vi "Database.Main-CheckStatus.vi"(8 "error in":errorcluster) -> (0 "error out":errorcluster)   [LabVIEW 2016]
uses:
  CheckStatusData.ctl
  Database.Main.Action.ctl
panel:
  in  "CheckStatusData":T1
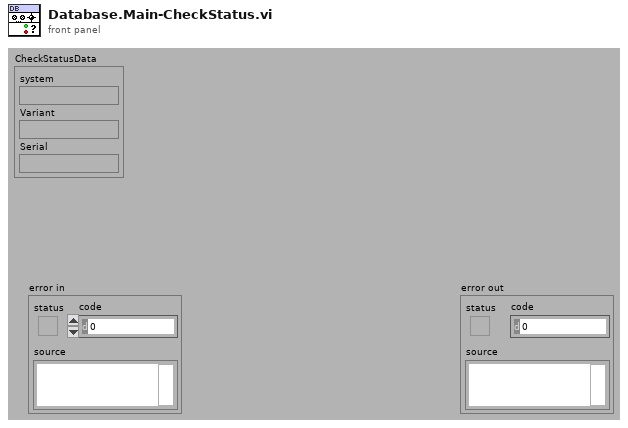
[diagram p1: front panel]
types:
  T1 = typedef "CheckStatusData.ctl" = cluster{"system":string, "Variant":string, "Serial":string}
  T2 = typedef "Database.Main.Action.ctl" = enum32{"idle", "constructor", "destructor", "--- DB ---", "Init", "Setup", "Select.Variant", "File.Export", "UpdateVariantFiles", "CheckStatus"}
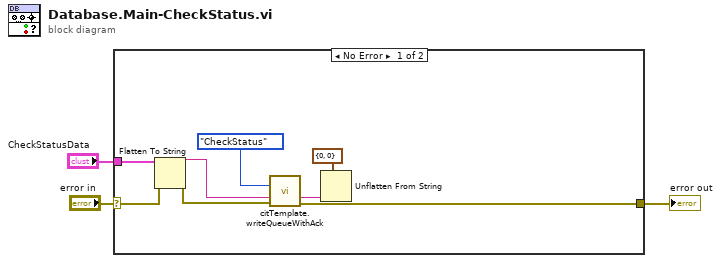
[diagram p0: block diagram]
diagram:
  n1 = case shown="No Error" "error in" {
    selector: "error in" -> [w8 w12]
    tunnel: [w11 w12] -> w2
    tunnel: "CheckStatusData" -> [w6 _]
    frame No Error {
      n2 = Flatten To String(anything=w6, error in (no error)=w8) -> (data string=w9:string, error out=w7:errorcluster)  [unwired: 2 in, 1 out]
      n3 = call "citTemplate.writeQueueWithAck.vi"("event in"=Database.Main.Action."CheckStatus" ("Action"), "(flatten) data in"=w9, "error in (no error)"=w7) -> ("notification data"=w5:string, "error out"=w11:errorcluster)  [unwired: 10 in, 1 out]
      n4 = Unflatten From String(type=cluster{u8, i8} {0, 0}, binary string=w5) -> ()  [unwired: 3 in, 3 out]
    }
    frame Error {
    }
  }
  "error out" <- w2
